vi "iFlex 2.0 .vi"(8 "error in":errorcluster, 11 "params":variant) -> (0 "error out":errorcluster)   [LabVIEW 2020]
uses:
  _Controls/iFlex.ctl
  Thorlabs/LSM_SDK/ThorConfocal.lvlib
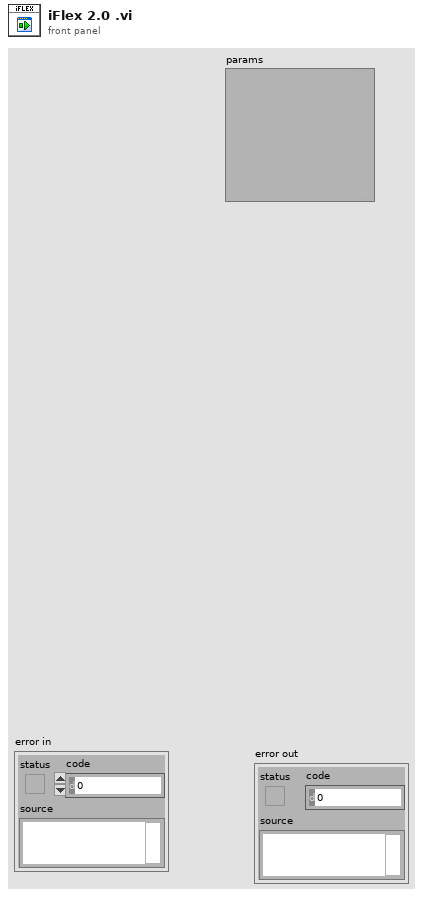
[diagram p1: front panel]
types:
  T1 = typedef "iFlex.ctl" = cluster{"561":dbl, "488":dbl, "Global Shutter":bool, "561 Shutter":bool}
  T2 = cluster{"iFlex Control":T1, "index of change":i32[]}
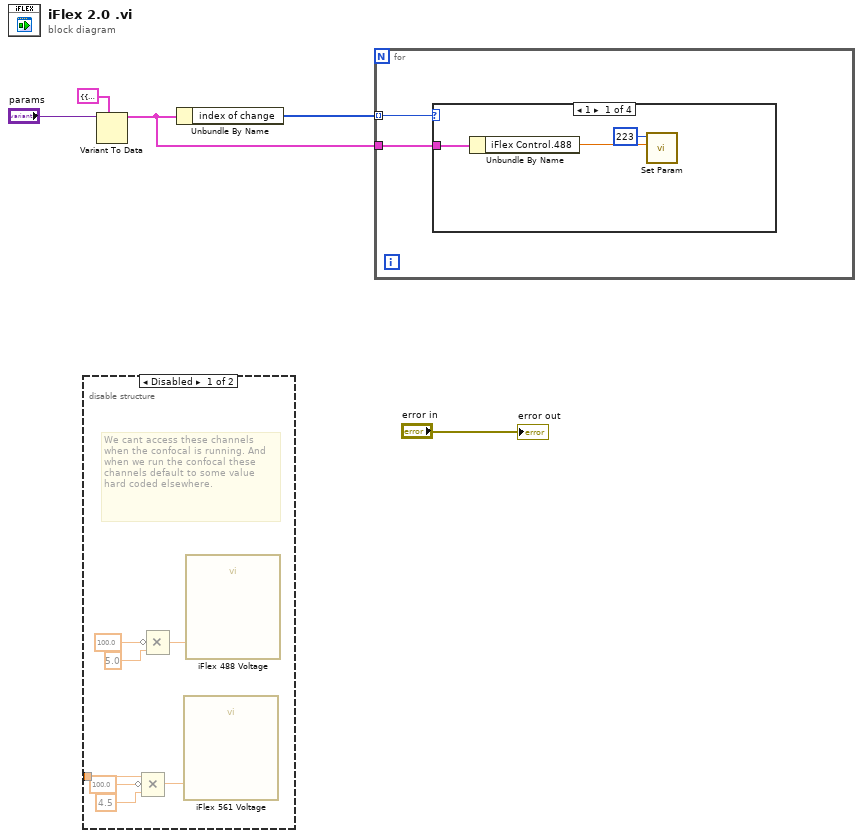
[diagram p0: block diagram]
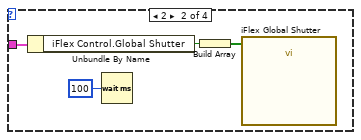
[diagram p2: hidden frame]
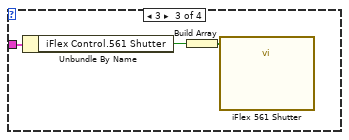
[diagram p3: hidden frame]
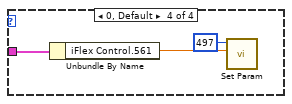
[diagram p4: hidden frame]
diagram:
  n1 = disable-structure shown="Disabled" {
    disable-tunnel: _ -> [w12 _]
    frame Disabled {
      # "We cant access these channels when the confocal is running. And when we run the confocal these channels default to some value hard coded elsewhere."
      n2 = Compound Arithmetic op=MULTIPLY(w12, invert 100.0 ("value"), 4.5 ("value")) -> (w6:dbl)
      n3 = Compound Arithmetic op=MULTIPLY(invert 100.0 ("value"), 5.0 ("value")) -> (w9:dbl)  [unwired: 1 in]
      n4 = call "iFlex 561 Voltage"("data"=w6) -> ()  [unwired: 17 in, 2 out]
      n5 = call "iFlex 488 Voltage"("data"=w9) -> ()  [unwired: 17 in, 2 out]
    }
    frame Enabled {
    }
  }
  n6 = Variant To Data(type=T2 {"iFlex Control"={"561"=0.0, "488"=0.0, "Global Shutter"=FALSE, "561 Shutter"=FALSE}, "index of change"=[]}, Variant="params") -> (data=w4:T2)  [unwired: 1 in, 1 out]
  n7 = Unbundle By Name(w4) -> ("index of change"=w1:i32[])
  n8 = for {
    tunnel: w1 -> [w14] mode=indexing
    tunnel: w4 -> [w13]
    n9 = case shown="1" w14 {
      tunnel: w13 -> [w16 w20 w23 w26]
      frame 1 {
        n10 = Unbundle By Name(w16) -> ("iFlex Control.488"=w15:dbl)
        n11 = call "Set Param.vi"("param"=w15, "paramID"=223) -> ()  [unwired: 4 in, 2 out]
      }
      frame 2 {
        n12 = Unbundle By Name(w20) -> ("iFlex Control.Global Shutter"=w19:bool)
        n13 = Wait (ms)(milliseconds to wait=u32 100) -> ()  [unwired: 1 out]
        n14 = Build Array(w19) -> (w21:bool[])
        n15 = call "iFlex Global Shutter"("data"=w21) -> ()  [unwired: 17 in, 2 out]
      }
      frame 3 {
        n16 = Unbundle By Name(w23) -> ("iFlex Control.561 Shutter"=w22:bool)
        n17 = Build Array(w22) -> (w24:bool[])
        n18 = call "iFlex 561 Shutter"("data"=w24) -> ()  [unwired: 17 in, 2 out]
      }
      frame 0, Default {
        n19 = Unbundle By Name(w26) -> ("iFlex Control.561"=w25:dbl)
        n20 = call "Set Param.vi"("param"=w25, "paramID"=497) -> ()  [unwired: 4 in, 2 out]
      }
    }
  }
  "error out" <- "error in"
